vi "nanocal -- nuclear schottky fit V8.vi"() -> ()   [LabVIEW 2021] (continued)
  out "string OUT":string="  \"IDS0158_210310_RAW_cal__ref_\" ->   <|    \"ζ\" -> 0.342934102355   ,  \"τ1\" -> 0.037912336866   ,  \"τS\" -> 0.322770587290   ,  \"τN\" -> 0.224517468406   ,  \"τC\" -> 0.000970428995   ,  \"κ0\" -> 0.000000000517   ,  \"mm1\" -> 0.000247395955   ,  \"mm2\" -> 0.021898106728   ,  \"mm3\" -> 0.751709056984   ,  \"T\" -> 0.120000000000   ,  \"B\" -> 12.000000000000   ,  \"θ\" -> 0.000000000000   ,  \"Reoff\" -> 0.000000000000   ,  \"Imoff\" -> 0.000000000000   ,  \"στ1\" -> 0.000893425914   ,  \"στS\" -> 0.002489408176   ,  \"στN\" -> 0.002611842121   ,  \"τ11 \" -> 0.000000000000   ,  \"τ12\" -> 0.000000000000   ,  \"τ22\" -> 0.000000000000   ,  \"τN1\" -> 0.000000000000   ,  \"τN2\" -> 0.000000000000   ,  \"σηlogτ1 \" -> 0.114569772809   ,  \"σηlogτS\" -> 0.007573309274   ,  \"σηlogτN\" -> 0.068166495911   ,  \"σlogτ1\" -> 0.023565572257   ,  \"σlogτS\" -> 0.007712623993   ,  \"σlogτN\" -> 0.011633135451   ,  \"σητ1\" -> 0.004343607821   ,  \"σητS \" -> 0.002444441482   ,  \"σητN\" -> 0.015304569092    |>   , \r\"IDS0158_210310_RAW_cal__sam_\" ->   <|    \"ζ\" -> 0.286336668596   ,  \"τ1\" -> 0.037477267671   ,  \"τS\" -> 0.354459287884   ,  \"τN\" -> 0.444916383639   ,  \"τC\" -> 0.001225600579   ,  \"κ0\" -> 0.000000000596   ,  \"mm1\" -> 0.000272242393   ,  \"mm2\" -> 0.016302418461   ,  \"mm3\" -> 1.050394445660   ,  \"T\" -> 0.120000000000   ,  \"B\" -> 12.000000000000   ,  \"θ\" -> 0.000000000000   ,  \"Reoff\" -> 0.000000000000   ,  \"Imoff\" -> 0.000000000000   ,  \"στ1\" -> 0.000000000000   ,  \"στS\" -> 0.000000000000   ,  \"στN\" -> 0.000000000000   ,  \"τ11 \" -> 0.000000000000   ,  \"τ12\" -> 0.000000000000   ,  \"τ22\" -> 0.000000000000   ,  \"τN1\" -> 0.000000000000   ,  \"τN2\" -> 0.000000000000   ,  \"σηlogτ1 \" -> 0.000000000000   ,  \"σηlogτS\" -> 0.000000000000   ,  \"σηlogτN\" -> 0.000000000000   ,  \"σlogτ1\" -> 0.000000000000   ,  \"σlogτS\" -> 0.000000000000   ,  \"σlogτN\" -> 0.000000000000   ,  \"σητ1\" -> 0.000000000000   ,  \"σητS \" -> 0.000000000000   ,  \"σητN\" -> 0.000000000000    |>   , \r\"IDS0159_210310_RAW_cal__ref_\" ->   <|    \"ζ\" -> 0.271761862806   ,  \"τ1\" -> 0.039955104592   ,  \"τS\" -> 0.227503722031   ,  \"τN\" -> 0.142080712192   ,  \"τC\" -> 0.000995450305   ,  \"κ0\" -> 0.000000000652   ,  \"mm1\" -> 0.000212140795   ,  \"mm2\" -> 0.023804196565   ,  \"mm3\" -> 0.486957606069   ,  \"T\" -> 0.150000000000   ,  \"B\" -> 12.000000000000   ,  \"θ\" -> 0.000000000000   ,  \"Reoff\" -> 0.000000000000   ,  \"Imoff\" -> 0.000000000000   ,  \"στ1\" -> 0.000698593116   ,  \"στS\" -> 0.001142949493   ,  \"στN\" -> 0.001230291496   ,  \"τ11 \" -> 0.000000000000   ,  \"τ12\" -> 0.000000000000   ,  \"τ22\" -> 0.000000000000   ,  \"τN1\" -> 0.000000000000   ,  \"τN2\" -> 0.000000000000   ,  \"σηlogτ1 \" -> 0.100498796621   ,  \"σηlogτS\" -> 0.005660617730   ,  \"σηlogτN\" -> 0.063140982058   ,  \"σlogτ1\" -> 0.017484452181   ,  \"σlogτS\" -> 0.005023871622   ,  \"σlogτN\" -> 0.008659102821   ,  \"σητ1\" -> 0.004015439930   ,  \"σητS \" -> 0.001287811603   ,  \"σητN\" -> 0.008971115699    |>   , \r\"IDS0159_210310_RAW_cal__sam_\" ->   <|    \"ζ\" -> 0.219100303741   ,  \"τ1\" -> 0.028643012604   ,  \"τS\" -> 0.279362928811   ,  \"τN\" -> 0.246156444058   ,  \"τC\" -> 0.001272401549   ,  \"κ0\" -> 0.000000000760   ,  \"mm1\" -> 0.000227975653   ,  \"mm2\" -> 0.014929571562   ,  \"mm3\" -> 0.655418694024   ,  \"T\" -> 0.150000000000   ,  \"B\" -> 12.000000000000   ,  \"θ\" -> 0.000000000000   ,  \"Reoff\" -> 0.000000000000   ,  \"Imoff\" -> 0.000000000000   ,  \"στ1\" -> 0.000000000000   ,  \"στS\" -> 0.000000000000   ,  \"στN\" -> 0.000000000000   ,  \"τ11 \" -> 0.000000000000   ,  \"τ12\" -> 0.000000000000   ,  \"τ22\" -> 0.000000000000   ,  \"τN1\" -> 0.000000000000   ,  \"τN2\" -> 0.000000000000   ,  \"σηlogτ1 \" -> 0.000000000000   ,  \"σηlogτS\" -> 0.000000000000   ,  \"σηlogτN\" -> 0.000000000000   ,  \"σlogτ1\" -> 0.000000000000   ,  \"σlogτS\" -> 0.000000000000   ,  \"σlogτN\" -> 0.000000000000   ,  \"σητ1\" -> 0.000000000000   ,  \"σητS \" -> 0.000000000000   ,  \"σητN\" -> 0.000000000000    |>   , \r\"IDS0160_210310_RAW_cal__ref_\" ->   <|    \"ζ\" -> 0.199613086212   ,  \"τ1\" -> 0.022193731398   ,  \"τS\" -> 0.116862561742   ,  \"τN\" -> 0.097247059130   ,  \"τC\" -> 0.001045881960   ,  \"κ0\" -> 0.000000000931   ,  \"mm1\" -> 0.000172948552   ,  \"mm2\" -> 0.011671612475   ,  \"mm3\" -> 0.268243755414   ,  \"T\" -> 0.180000000000   ,  \"B\" -> 12.000000000000   ,  \"θ\" -> 0.000000000000   ,  \"Reoff\" -> 0.000000000000   ,  \"Imoff\" -> 0.000000000000   ,  \"στ1\" -> 0.000089856815   ,  \"στS\" -> 0.000165029214   ,  \"στN\" -> 0.000188286128   ,  \"τ11 \" -> 0.000000000000   ,  \"τ12\" -> 0.000000000000   ,  \"τ22\" -> 0.000000000000   ,  \"τN1\" -> 0.000000000000   ,  \"τN2\" -> 0.000000000000   ,  \"σηlogτ1 \" -> 0.093550953866   ,  \"σηlogτS\" -> 0.006075230131   ,  \"σηlogτN\" -> 0.064015363974   ,  \"σlogτ1\" -> 0.004048747519   ,  \"σlogτS\" -> 0.001412164955   ,  \"σlogτN\" -> 0.001936162698   ,  \"σητ1\" -> 0.002076244742   ,  \"σητS \" -> 0.000709966956   ,  \"σητN\" -> 0.006225305886    |>   , \r\"IDS0160_210310_RAW_cal__sam_\" ->   <|    \"ζ\" -> 0.170488637524   ,  \"τ1\" -> 0.029234231120   ,  \"τS\" -> 0.149095458227   ,  \"τN\" -> 0.151792620275   ,  \"τC\" -> 0.001113424175   ,  \"κ0\" -> 0.000000001042   ,  \"mm1\" -> 0.000161291869   ,  \"mm2\" -> 0.013922632736   ,  \"mm3\" -> 0.368449807743   ,  \"T\" -> 0.180000000000   ,  \"B\" -> 12.000000000000   ,  \"θ\" -> 0.000000000000   ,  \"Reoff\" -> 0.000000000000   ,  \"Imoff\" -> 0.000000000000   ,  \"στ1\" -> 0.000000000000   ,  \"στS\" -> 0.000000000000   ,  \"στN\" -> 0.000000000000   ,  \"τ11 \" -> 0.000000000000   ,  \"τ12\" -> 0.000000000000   ,  \"τ22\" -> 0.000000000000   ,  \"τN1\" -> 0.000000000000   ,  \"τN2\" -> 0.000000000000   ,  \"σηlogτ1 \" -> 0.000000000000   ,  \"σηlogτS\" -> 0.000000000000   ,  \"σηlogτN\" -> 0.000000000000   ,  \"σlogτ1\" -> 0.000000000000   ,  \"σlogτS\" -> 0.000000000000   ,  \"σlogτN\" -> 0.000000000000   ,  \"σητ1\" -> 0.000000000000   ,  \"σητS \" -> 0.000000000000   ,  \"σητN\" -> 0.000000000000    |>   , \r\"IDS0161_210310_RAW_cal__ref_\" ->   <|    \"ζ\" -> 0.155485326727   ,  \"τ1\" -> 0.024589160211   ,  \"τS\" -> 0.103187251839   ,  \"τN\" -> 0.059327264902   ,  \"τC\" -> 0.001362397594   ,  \"κ0\" -> 0.000000001075   ,  \"mm1\" -> 0.000181522487   ,  \"mm2\" -> 0.014905594718   ,  \"mm3\" -> 0.198647580074   ,  \"T\" -> 0.200000000000   ,  \"B\" -> 12.000000000000   ,  \"θ\" -> 0.000000000000   ,  \"Reoff\" -> 0.000000000000   ,  \"Imoff\" -> 0.000000000000   ,  \"στ1\" -> 0.000106824093   ,  \"στS\" -> 0.000114207069   ,  \"στN\" -> 0.000127738509   ,  \"τ11 \" -> 0.000000000000   ,  \"τ12\" -> 0.000000000000   ,  \"τ22\" -> 0.000000000000   ,  \"τN1\" -> 0.000000000000   ,  \"τN2\" -> 0.000000000000   ,  \"σηlogτ1 \" -> 0.086294510505   ,  \"σηlogτS\" -> 0.004144737065   ,  \"σηlogτN\" -> 0.058529518145   ,  \"σlogτ1\" -> 0.004344357106   ,  \"σlogτS\" -> 0.001106794371   ,  \"σlogτN\" -> 0.002153116435   ,  \"σητ1\" -> 0.002121909544   ,  \"σητS \" -> 0.000427684027   ,  \"σητN\" -> 0.003472396228    |>   , \r\"IDS0161_210310_RAW_cal__sam_\" ->   <|    \"ζ\" -> 0.130531197151   ,  \"τ1\" -> 0.025704482770   ,  \"τS\" -> 0.129606657196   ,  \"τN\" -> 0.091602369165   ,  \"τC\" -> 0.001441379995   ,  \"κ0\" -> 0.000000001211   ,  \"mm1\" -> 0.000164978070   ,  \"mm2\" -> 0.014468182937   ,  \"mm3\" -> 0.262596407151   ,  \"T\" -> 0.200000000000   ,  \"B\" -> 12.000000000000   ,  \"θ\" -> 0.000000000000   ,  \"Reoff\" -> 0.000000000000   ,  \"Imoff\" -> 0.000000000000   ,  \"στ1\" -> 0.000000000000   ,  \"στS\" -> 0.000000000000   ,  \"στN\" -> 0.000000000000   ,  \"τ11 \" -> 0.000000000000   ,  \"τ12\" -> 0.000000000000   ,  \"τ22\" -> 0.000000000000   ,  \"τN1\" -> 0.000000000000   ,  \"τN2\" -> 0.000000000000   ,  \"σηlogτ1 \" -> 0.000000000000   ,  \"σηlogτS\" -> 0.000000000000   ,  \"σηlogτN\" -> 0.000000000000   ,  \"σlogτ1\" -> 0.000000000000   ,  \"σlogτS\" -> 0.000000000000   ,  \"σlogτN\" -> 0.000000000000   ,  \"σητ1\" -> 0.000000000000   ,  \"σητS \" -> 0.000000000000   ,  \"σητN\" -> 0.000000000000    |>   , \r\"IDS0162_210310_RAW_cal__ref_\" ->   <|    \"ζ\" -> 0.085932974943   ,  \"τ1\" -> 0.018822470857   ,  \"τS\" -> 0.068810147904   ,  \"τN\" -> 0.024216831887   ,  \"τC\" -> 0.001953952621   ,  \"κ0\" -> 0.000000001388   ,  \"mm1\" -> 0.000150968751   ,  \"mm2\" -> 0.013294741414   ,  \"mm3\" -> 0.108351778227   ,  \"T\" -> 0.250000000000   ,  \"B\" -> 12.000000000000   ,  \"θ\" -> 0.000000000000   ,  \"Reoff\" -> 0.000000000000   ,  \"Imoff\" -> 0.000000000000   ,  \"στ1\" -> 0.000058321163   ,  \"στS\" -> 0.000035049706   ,  \"στN\" -> 0.000037861271   ,  \"τ11 \" -> 0.000000000000   ,  \"τ12\" -> 0.000000000000   ,  \"τ22\" -> 0.000000000000   ,  \"τN1\" -> 0.000000000000   ,  \"τN2\" -> 0.000000000000   ,  \"σηlogτ1 \" -> 0.080513059924   ,  \"σηlogτS\" -> 0.002518022810   ,  \"σηlogτN\" -> 0.054257654253   ,  \"σlogτ1\" -> 0.003098486056   ,  \"σlogτS\" -> 0.000509368271   ,  \"σlogτN\" -> 0.001563427918   ,  \"σητ1\" -> 0.001515454724   ,  \"σητS \" -> 0.000173265522   ,  \"σητN\" -> 0.001313948492    |>   , \r\"IDS0162_210310_RAW_cal__sam_\" ->   <|    \"ζ\" -> 0.078258046754   ,  \"τ1\" -> 0.028009840731   ,  \"τS\" -> 0.092122038762   ,  \"τN\" -> 0.030129595899   ,  \"τC\" -> 0.001641062244   ,  \"κ0\" -> 0.000000001543   ,  \"mm1\" -> 0.000117303440   ,  \"mm2\" -> 0.019983073008   ,  \"mm3\" -> 0.141369335330   ,  \"T\" -> 0.250000000000   ,  \"B\" -> 12.000000000000   ,  \"θ\" -> 0.000000000000   ,  \"Reoff\" -> 0.000000000000   ,  \"Imoff\" -> 0.000000000000   ,  \"στ1\" -> 0.000000000000   ,  \"στS\" -> 0.000000000000   ,  \"στN\" -> 0.000000000000   ,  \"τ11 \" -> 0.000000000000   ,  \"τ12\" -> 0.000000000000   ,  \"τ22\" -> 0.000000000000   ,  \"τN1\" -> 0.000000000000   ,  \"τN2\" -> 0.000000000000   ,  \"σηlogτ1 \" -> 0.000000000000   ,  \"σηlogτS\" -> 0.000000000000   ,  \"σηlogτN\" -> 0.000000000000   ,  \"σlogτ1\" -> 0.000000000000   ,  \"σlogτS\" -> 0.000000000000   ,  \"σlogτN\" -> 0.000000000000   ,  \"σητ1\" -> 0.000000000000   ,  \"σητS \" -> 0.000000000000   ,  \"σητN\" -> 0.000000000000    |>   , \r\"IDS0163_210310_RAW_cal__ref_\" ->   <|    \"ζ\" -> 0.058825748663   ,  \"τ1\" -> 0.015012107932   ,  \"τS\" -> 0.052128918860   ,  \"τN\" -> 0.012953217864   ,  \"τC\" -> 0.002393557537   ,  \"κ0\" -> 0.000000001766   ,  \"mm1\" -> 0.000127725677   ,  \"mm2\" -> 0.011559700576   ,  \"mm3\" -> 0.074628881357   ,  \"T\" -> 0.300000000000   ,  \"B\" -> 12.000000000000   ,  \"θ\" -> 0.000000000000   ,  \"Reoff\" -> 0.000000000000   ,  \"Imoff\" -> 0.000000000000   ,  \"στ1\" -> 0.000023064935   ,  \"στS\" -> 0.000009573131   ,  \"στN\" -> 0.000010092664   ,  \"τ11 \" -> 0.000000000000   ,  \"τ12\" -> 0.000000000000   ,  \"τ22\" -> 0.000000000000   ,  \"τN1\" -> 0.000000000000   ,  \"τN2\" -> 0.000000000000   ,  \"σηlogτ1 \" -> 0.078709092172   ,  \"σηlogτS\" -> 0.001802886041   ,  \"σηlogτN\" -> 0.052574057148   ,  \"σlogτ1\" -> 0.001536422126   ,  \"σlogτS\" -> 0.000183643382   ,  \"σlogτN\" -> 0.000779162669   ,  \"σητ1\" -> 0.001181589387   ,  \"σητS \" -> 0.000093982500   ,  \"σητN\" -> 0.000681003216    |>   , \r\"IDS0163_210310_RAW_cal__sam_\" ->   <|    \"ζ\" -> 0.054088186012   ,  \"τ1\" -> 0.023838802615   ,  \"τS\" -> 0.069079396629   ,  \"τN\" -> 0.016435267456   ,  \"τC\" -> 0.002025071743   ,  \"κ0\" -> 0.000000001955   ,  \"mm1\" -> 0.000101234646   ,  \"mm2\" -> 0.018244822177   ,  \"mm3\" -> 0.097657814678   ,  \"T\" -> 0.300000000000   ,  \"B\" -> 12.000000000000   ,  \"θ\" -> 0.000000000000   ,  \"Reoff\" -> 0.000000000000   ,  \"Imoff\" -> 0.000000000000   ,  \"στ1\" -> 0.000000000000   ,  \"στS\" -> 0.000000000000   ,  \"στN\" -> 0.000000000000   ,  \"τ11 \" -> 0.000000000000   ,  \"τ12\" -> 0.000000000000   ,  \"τ22\" -> 0.000000000000   ,  \"τN1\" -> 0.000000000000   ,  \"τN2\" -> 0.000000000000   ,  \"σηlogτ1 \" -> 0.000000000000   ,  \"σηlogτS\" -> 0.000000000000   ,  \"σηlogτN\" -> 0.000000000000   ,  \"σlogτ1\" -> 0.000000000000   ,  \"σlogτS\" -> 0.000000000000   ,  \"σlogτN\" -> 0.000000000000   ,  \"σητ1\" -> 0.000000000000   ,  \"σητS \" -> 0.000000000000   ,  \"σητN\" -> 0.000000000000    |>   , \r\"IDS0164_210310_RAW_cal__ref_\" ->   <|    \"ζ\" -> 0.042805749253   ,  \"τ1\" -> 0.013206199214   ,  \"τS\" -> 0.042245691100   ,  \"τN\" -> 0.007144228501   ,  \"τC\" -> 0.002899499229   ,  \"κ0\" -> 0.000000002181   ,  \"mm1\" -> 0.000111927858   ,  \"mm2\" -> 0.010938028304   ,  \"mm3\" -> 0.056559834396   ,  \"T\" -> 0.360000000000   ,  \"B\" -> 12.000000000000   ,  \"θ\" -> 0.000000000000   ,  \"Reoff\" -> 0.000000000000   ,  \"Imoff\" -> 0.000000000000   ,  \"στ1\" -> 0.000012292384   ,  \"στS\" -> 0.000003241338   ,  \"στN\" -> 0.000003368378   ,  \"τ11 \" -> 0.000000000000   ,  \"τ12\" -> 0.000000000000   ,  \"τ22\" -> 0.000000000000   ,  \"τN1\" -> 0.000000000000   ,  \"τN2\" -> 0.000000000000   ,  \"σηlogτ1 \" -> 0.075974060792   ,  \"σηlogτS\" -> 0.001194926073   ,  \"σηlogτN\" -> 0.051138297484   ,  \"σlogτ1\" -> 0.000930804037   ,  \"σlogτS\" -> 0.000076725884   ,  \"σlogτN\" -> 0.000471482447   ,  \"σητ1\" -> 0.001003328582   ,  \"σητS \" -> 0.000050480478   ,  \"σητN\" -> 0.000365343682    |>   , \r\"IDS0164_210310_RAW_cal__sam_\" ->   <|    \"ζ\" -> 0.039314966212   ,  \"τ1\" -> 0.020712803909   ,  \"τS\" -> 0.055413767550   ,  \"τN\" -> 0.008474403424   ,  \"τC\" -> 0.002674063387   ,  \"κ0\" -> 0.000000002415   ,  \"mm1\" -> 0.000096818147   ,  \"mm2\" -> 0.017190811405   ,  \"mm3\" -> 0.072499170001   ,  \"T\" -> 0.360000000000   ,  \"B\" -> 12.000000000000   ,  \"θ\" -> 0.000000000000   ,  \"Reoff\" -> 0.000000000000   ,  \"Imoff\" -> 0.000000000000   ,  \"στ1\" -> 0.000000000000   ,  \"στS\" -> 0.000000000000   ,  \"στN\" -> 0.000000000000   ,  \"τ11 \" -> 0.000000000000   ,  \"τ12\" -> 0.000000000000   ,  \"τ22\" -> 0.000000000000   ,  \"τN1\" -> 0.000000000000   ,  \"τN2\" -> 0.000000000000   ,  \"σηlogτ1 \" -> 0.000000000000   ,  \"σηlogτS\" -> 0.000000000000   ,  \"σηlogτN\" -> 0.000000000000   ,  \"σlogτ1\" -> 0.000000000000   ,  \"σlogτS\" -> 0.000000000000   ,  \"σlogτN\" -> 0.000000000000   ,  \"σητ1\" -> 0.000000000000   ,  \"σητS \" -> 0.000000000000   ,  \"σητN\" -> 0.000000000000    |>   , \r\"IDS0165_210310_RAW_cal__ref_\" ->   <|    \"ζ\" -> 0.032274621211   ,  \"τ1\" -> 0.011425652621   ,  \"τS\" -> 0.034817148793   ,  \"τN\" -> 0.004293407669   ,  \"τC\" -> 0.003209213512   ,  \"κ0\" -> 0.000000002697   ,  \"mm1\" -> 0.000092323212   ,  \"mm2\" -> 0.009918344751   ,  \"mm3\" -> 0.044997033026   ,  \"T\" -> 0.430000000000   ,  \"B\" -> 12.000000000000   ,  \"θ\" -> 0.000000000000   ,  \"Reoff\" -> 0.000000000000   ,  \"Imoff\" -> 0.000000000000   ,  \"στ1\" -> 0.000021533973   ,  \"στS\" -> 0.000003977444   ,  \"στN\" -> 0.000004093454   ,  \"τ11 \" -> 0.000000000000   ,  \"τ12\" -> 0.000000000000   ,  \"τ22\" -> 0.000000000000   ,  \"τN1\" -> 0.000000000000   ,  \"τN2\" -> 0.000000000000   ,  \"σηlogτ1 \" -> 0.074657261466   ,  \"σηlogτS\" -> 0.000861446772   ,  \"σηlogτN\" -> 0.050403269276   ,  \"σlogτ1\" -> 0.001884703953   ,  \"σlogτS\" -> 0.000114238081   ,  \"σlogτN\" -> 0.000953427722   ,  \"σητ1\" -> 0.000853007935   ,  \"σητS \" -> 0.000029993120   ,  \"σητN\" -> 0.000216401783    |>   , \r\"IDS0165_210310_RAW_cal__sam_\" ->   <|    \"ζ\" -> 0.031945976845   ,  \"τ1\" -> 0.019000922826   ,  \"τS\" -> 0.045624146388   ,  \"τN\" -> 0.005314716063   ,  \"τC\" -> 0.002488383471   ,  \"κ0\" -> 0.000000002954   ,  \"mm1\" -> 0.000073272643   ,  \"mm2\" -> 0.016306894362   ,  \"mm3\" -> 0.057675293464   ,  \"T\" -> 0.430000000000   ,  \"B\" -> 12.000000000000   ,  \"θ\" -> 0.000000000000   ,  \"Reoff\" -> 0.000000000000   ,  \"Imoff\" -> 0.000000000000   ,  \"στ1\" -> 0.000000000000   ,  \"στS\" -> 0.000000000000   ,  \"στN\" -> 0.000000000000   ,  \"τ11 \" -> 0.000000000000   ,  \"τ12\" -> 0.000000000000   ,  \"τ22\" -> 0.000000000000   ,  \"τN1\" -> 0.000000000000   ,  \"τN2\" -> 0.000000000000   ,  \"σηlogτ1 \" -> 0.000000000000   ,  \"σηlogτS\" -> 0.000000000000   ,  \"σηlogτN\" -> 0.000000000000   ,  \"σlogτ1\" -> 0.000000000000   ,  \"σlogτS\" -> 0.000000000000   ,  \"σlogτN\" -> 0.000000000000   ,  \"σητ1\" -> 0.000000000000   ,  \"σητS \" -> 0.000000000000   ,  \"σητN\" -> 0.000000000000    |>   , \r\"IDS0166_210310_RAW_cal__ref_\" ->   <|    \"ζ\" -> 0.024856483242   ,  \"τ1\" -> 0.010695421072   ,  \"τS\" -> 0.028584689386   ,  \"τN\" -> 0.002299338912   ,  \"τC\" -> 0.003707358018   ,  \"κ0\" -> 0.000000003388   ,  \"mm1\" -> 0.000080004626   ,  \"mm2\" -> 0.009710607688   ,  \"mm3\" -> 0.036263863406   ,  \"T\" -> 0.520000000000   ,  \"B\" -> 12.000000000000   ,  \"θ\" -> 0.000000000000   ,  \"Reoff\" -> 0.000000000000   ,  \"Imoff\" -> 0.000000000000   ,  \"στ1\" -> 0.000044725972   ,  \"στS\" -> 0.000004660348   ,  \"στN\" -> 0.000004819065   ,  \"τ11 \" -> 0.000000000000   ,  \"τ12\" -> 0.000000000000   ,  \"τ22\" -> 0.000000000000   ,  \"τN1\" -> 0.000000000000   ,  \"τN2\" -> 0.000000000000   ,  \"σηlogτ1 \" -> 0.070445110801   ,  \"σηlogτS\" -> 0.000510235434   ,  \"σηlogτN\" -> 0.049344443023   ,  \"σlogτ1\" -> 0.004181786915   ,  \"σlogτS\" -> 0.000163036495   ,  \"σlogτN\" -> 0.002095848078   ,  \"σητ1\" -> 0.000753440123   ,  \"σητS \" -> 0.000014584921   ,  \"σητN\" -> 0.000113459598    |>   , \r\"IDS0166_210310_RAW_cal__sam_\" ->   <|    \"ζ\" -> 0.023031239946   ,  \"τ1\" -> 0.018268814012   ,  \"τS\" -> 0.037269400776   ,  \"τN\" -> 0.002696792890   ,  \"τC\" -> 0.003257395394   ,  \"κ0\" -> 0.000000003720   ,  \"mm1\" -> 0.000067670174   ,  \"mm2\" -> 0.016445281937   ,  \"mm3\" -> 0.045899921957   ,  \"T\" -> 0.520000000000   ,  \"B\" -> 12.000000000000   ,  \"θ\" -> 0.000000000000   ,  \"Reoff\" -> 0.000000000000   ,  \"Imoff\" -> 0.000000000000   ,  \"στ1\" -> 0.000000000000   ,  \"στS\" -> 0.000000000000   ,  \"στN\" -> 0.000000000000   ,  \"τ11 \" -> 0.000000000000   ,  \"τ12\" -> 0.000000000000   ,  \"τ22\" -> 0.000000000000   ,  \"τN1\" -> 0.000000000000   ,  \"τN2\" -> 0.000000000000   ,  \"σηlogτ1 \" -> 0.000000000000   ,  \"σηlogτS\" -> 0.000000000000   ,  \"σηlogτN\" -> 0.000000000000   ,  \"σlogτ1\" -> 0.000000000000   ,  \"σlogτS\" -> 0.000000000000   ,  \"σlogτN\" -> 0.000000000000   ,  \"σητ1\" -> 0.000000000000   ,  \"σητS \" -> 0.000000000000   ,  \"σητN\" -> 0.000000000000    |>   , \r\"IDS0167_210310_RAW_cal__ref_\" ->   <|    \"ζ\" -> 0.023755086775   ,  \"τ1\" -> 0.012442537684   ,  \"τS\" -> 0.025226466021   ,  \"τN\" -> 0.001327754553   ,  \"τC\" -> 0.003535029288   ,  \"κ0\" -> 0.000000003992   ,  \"mm1\" -> 0.000072325961   ,  \"mm2\" -> 0.011557286901   ,  \"mm3\" -> 0.031532972498   ,  \"T\" -> 0.620000000000   ,  \"B\" -> 12.000000000000   ,  \"θ\" -> 0.000000000000   ,  \"Reoff\" -> 0.000000000000   ,  \"Imoff\" -> 0.000000000000   ,  \"στ1\" -> 0.000121120374   ,  \"στS\" -> 0.000005759367   ,  \"στN\" -> 0.000006380048   ,  \"τ11 \" -> 0.000000000000   ,  \"τ12\" -> 0.000000000000   ,  \"τ22\" -> 0.000000000000   ,  \"τN1\" -> 0.000000000000   ,  \"τN2\" -> 0.000000000000   ,  \"σηlogτ1 \" -> 0.060087437694   ,  \"σηlogτS\" -> 0.000239286620   ,  \"σηlogτN\" -> 0.047627856995   ,  \"σlogτ1\" -> 0.009734378741   ,  \"σlogτS\" -> 0.000228306534   ,  \"σlogτN\" -> 0.004805140830   ,  \"σητ1\" -> 0.000747640208   ,  \"σητS \" -> 0.000006036356   ,  \"σητN\" -> 0.000063238104    |>   , \r\"IDS0167_210310_RAW_cal__sam_\" ->   <|    \"ζ\" -> 0.019920170845   ,  \"τ1\" -> 0.016368892412   ,  \"τS\" -> 0.030579536580   ,  \"τN\" -> 0.001736017565   ,  \"τC\" -> 0.004971418152   ,  \"κ0\" -> 0.000000004410   ,  \"mm1\" -> 0.000083939556   ,  \"mm2\" -> 0.015095997595   ,  \"mm3\" -> 0.039119658918   ,  \"T\" -> 0.620000000000   ,  \"B\" -> 12.000000000000   ,  \"θ\" -> 0.000000000000   ,  \"Reoff\" -> 0.000000000000   ,  \"Imoff\" -> 0.000000000000   ,  \"στ1\" -> 0.000000000000   ,  \"στS\" -> 0.000000000000   ,  \"στN\" -> 0.000000000000   ,  \"τ11 \" -> 0.000000000000   ,  \"τ12\" -> 0.000000000000   ,  \"τ22\" -> 0.000000000000   ,  \"τN1\" -> 0.000000000000   ,  \"τN2\" -> 0.000000000000   ,  \"σηlogτ1 \" -> 0.000000000000   ,  \"σηlogτS\" -> 0.000000000000   ,  \"σηlogτN\" -> 0.000000000000   ,  \"σlogτ1\" -> 0.000000000000   ,  \"σlogτS\" -> 0.000000000000   ,  \"σlogτN\" -> 0.000000000000   ,  \"σητ1\" -> 0.000000000000   ,  \"σητS \" -> 0.000000000000   ,  \"σητN\" -> 0.000000000000    |>   , \r\"IDS0168_210310_RAW_cal__ref_\" ->   <|    \"ζ\" -> 0.018175201883   ,  \"τ1\" -> 0.013383195137   ,  \"τS\" -> 0.017675939869   ,  \"τN\" -> 0.000584160710   ,  \"τC\" -> 0.005568397021   ,  \"κ0\" -> 0.000000005579   ,  \"mm1\" -> 0.000076155273   ,  \"mm2\" -> 0.012686054664   ,  \"mm3\" -> 0.024781363815   ,  \"T\" -> 0.810000000000   ,  \"B\" -> 12.000000000000   ,  \"θ\" -> 0.000000000000   ,  \"Reoff\" -> 0.000000000000   ,  \"Imoff\" -> 0.000000000000   ,  \"στ1\" -> 0.000105801087   ,  \"στS\" -> 0.000001832616   ,  \"στN\" -> 0.000002314917   ,  \"τ11 \" -> 0.000000000000   ,  \"τ12\" -> 0.000000000000   ,  \"τ22\" -> 0.000000000000   ,  \"τN1\" -> 0.000000000000   ,  \"τN2\" -> 0.000000000000   ,  \"σηlogτ1 \" -> 0.050518101739   ,  \"σηlogτS\" -> 0.000100664856   ,  \"σηlogτN\" -> 0.045919539288   ,  \"σlogτ1\" -> 0.007905517739   ,  \"σlogτS\" -> 0.000103678550   ,  \"σlogτN\" -> 0.003962808035   ,  \"σητ1\" -> 0.000676093614   ,  \"σητS \" -> 0.000001779346   ,  \"σητN\" -> 0.000026824391    |>   , \r\"IDS0168_210310_RAW_cal__sam_\" ->   <|    \"ζ\" -> 0.017558473054   ,  \"τ1\" -> 0.014545104284   ,  \"τS\" -> 0.022979681288   ,  \"τN\" -> 0.000840829385   ,  \"τC\" -> 0.005228030240   ,  \"κ0\" -> 0.000000006068   ,  \"mm1\" -> 0.000073916527   ,  \"mm2\" -> 0.013750428362   ,  \"mm3\" -> 0.030187552103   ,  \"T\" -> 0.810000000000   ,  \"B\" -> 12.000000000000   ,  \"θ\" -> 0.000000000000   ,  \"Reoff\" -> 0.000000000000   ,  \"Imoff\" -> 0.000000000000   ,  \"στ1\" -> 0.000000000000   ,  \"στS\" -> 0.000000000000   ,  \"στN\" -> 0.000000000000   ,  \"τ11 \" -> 0.000000000000   ,  \"τ12\" -> 0.000000000000   ,  \"τ22\" -> 0.000000000000   ,  \"τN1\" -> 0.000000000000   ,  \"τN2\" -> 0.000000000000   ,  \"σηlogτ1 \" -> 0.000000000000   ,  \"σηlogτS\" -> 0.000000000000   ,  \"σηlogτN\" -> 0.000000000000   ,  \"σlogτ1\" -> 0.000000000000   ,  \"σlogτS\" -> 0.000000000000   ,  \"σlogτN\" -> 0.000000000000   ,  \"σητ1\" -> 0.000000000000   ,  \"σητS \" -> 0.000000000000   ,  \"σητN\" -> 0.000000000000    |>   , \r\"IDS0169_210310_RAW_cal__ref_\" ->   <|    \"ζ\" -> 0.019957179421   ,  \"τ1\" -> 0.013979356395   ,  \"τS\" -> 0.014979933171   ,  \"τN\" -> 0.000246381668   ,  \"τC\" -> 0.003917957379   ,  \"κ0\" -> 0.000000007787   ,  \"mm1\" -> 0.000061209589   ,  \"mm2\" -> 0.013393834195   ,  \"mm3\" -> 0.019972459127   ,  \"T\" -> 1.120000000000   ,  \"B\" -> 12.000000000000   ,  \"θ\" -> 0.000000000000   ,  \"Reoff\" -> -604081.632653061067   ,  \"Imoff\" -> 0.000000000000   ,  \"στ1\" -> 0.016865078301   ,  \"στS\" -> 0.000159497722   ,  \"στN\" -> 0.007867947468   ,  \"τ11 \" -> 0.000000000000   ,  \"τ12\" -> 0.000000000000   ,  \"τ22\" -> 0.000000000000   ,  \"τN1\" -> 0.000000000000   ,  \"τN2\" -> 0.000000000000   ,  \"σηlogτ1 \" -> 0.000000000000   ,  \"σηlogτS\" -> 0.000000000000   ,  \"σηlogτN\" -> 0.000000000000   ,  \"σlogτ1\" -> 0.000000000000   ,  \"σlogτS\" -> 0.000000000000   ,  \"σlogτN\" -> 0.000000000000   ,  \"σητ1\" -> 0.000000000000   ,  \"σητS \" -> 0.000000000000   ,  \"σητN\" -> 0.000000000000    |>   , \r\"IDS0169_210310_RAW_cal__sam_\" ->   <|    \"ζ\" -> 0.011916480594   ,  \"τ1\" -> 0.012551282481   ,  \"τS\" -> 0.018233218660   ,  \"τN\" -> 0.000345702746   ,  \"τC\" -> 0.004699451527   ,  \"κ0\" -> 0.000000008451   ,  \"mm1\" -> 0.000044190864   ,  \"mm2\" -> 0.012162820727   ,  \"mm3\" -> 0.023844039179   ,  \"T\" -> 1.120000000000   ,  \"B\" -> 12.000000000000   ,  \"θ\" -> 0.000000000000   ,  \"Reoff\" -> 0.000000000000   ,  \"Imoff\" -> 0.000000000000   ,  \"στ1\" -> 0.000000000000   ,  \"στS\" -> 0.000000000000   ,  \"στN\" -> 0.000000000000   ,  \"τ11 \" -> 0.000000000000   ,  \"τ12\" -> 0.000000000000   ,  \"τ22\" -> 0.000000000000   ,  \"τN1\" -> 0.000000000000   ,  \"τN2\" -> 0.000000000000   ,  \"σηlogτ1 \" -> 0.000000000000   ,  \"σηlogτS\" -> 0.000000000000   ,  \"σηlogτN\" -> 0.000000000000   ,  \"σlogτ1\" -> 0.000000000000   ,  \"σlogτS\" -> 0.000000000000   ,  \"σlogτN\" -> 0.000000000000   ,  \"σητ1\" -> 0.000000000000   ,  \"σητS \" -> 0.000000000000   ,  \"σητN\" -> 0.000000000000    |>   , \r\"IDS0170_210310_RAW_cal__ref_\" ->   <|    \"ζ\" -> 0.020917521423   ,  \"τ1\" -> 0.014571936752   ,  \"τS\" -> 0.010774968577   ,  \"τN\" -> 0.000062073801   ,  \"τC\" -> 0.003888097391   ,  \"κ0\" -> 0.000000012613   ,  \"mm1\" -> 0.000059093319   ,  \"mm2\" -> 0.013758745196   ,  \"mm3\" -> 0.015705922073   ,  \"T\" -> 1.800000000000   ,  \"B\" -> 12.000000000000   ,  \"θ\" -> 0.000000000000   ,  \"Reoff\" -> -530612.244897959054   ,  \"Imoff\" -> 0.000000000000   ,  \"στ1\" -> 0.055735786157   ,  \"στS\" -> 0.000157216248   ,  \"στN\" -> 0.024225134913   ,  \"τ11 \" -> 0.000000000000   ,  \"τ12\" -> 0.000000000000   ,  \"τ22\" -> 0.000000000000   ,  \"τN1\" -> 0.000000000000   ,  \"τN2\" -> 0.000000000000   ,  \"σηlogτ1 \" -> 0.000000000000   ,  \"σηlogτS\" -> 0.000000000000   ,  \"σηlogτN\" -> 0.000000000000   ,  \"σlogτ1\" -> 0.000000000000   ,  \"σlogτS\" -> 0.000000000000   ,  \"σlogτN\" -> 0.000000000000   ,  \"σητ1\" -> 0.000000000000   ,  \"σητS \" -> 0.000000000000   ,  \"σητN\" -> 0.000000000000    |>   , \r\"IDS0170_210310_RAW_cal__sam_\" ->   <|    \"ζ\" -> 0.012831327568   ,  \"τ1\" -> 0.013315909415   ,  \"τS\" -> 0.012590836847   ,  \"τN\" -> 0.000065003013   ,  \"τC\" -> 0.005276356243   ,  \"κ0\" -> 0.000000013610   ,  \"mm1\" -> 0.000047406274   ,  \"mm2\" -> 0.013137605540   ,  \"mm3\" -> 0.018225484932   ,  \"T\" -> 1.800000000000   ,  \"B\" -> 12.000000000000   ,  \"θ\" -> 0.000000000000   ,  \"Reoff\" -> 0.000000000000   ,  \"Imoff\" -> 0.000000000000   ,  \"στ1\" -> 0.000000000000   ,  \"στS\" -> 0.000000000000   ,  \"στN\" -> 0.000000000000   ,  \"τ11 \" -> 0.000000000000   ,  \"τ12\" -> 0.000000000000   ,  \"τ22\" -> 0.000000000000   ,  \"τN1\" -> 0.000000000000   ,  \"τN2\" -> 0.000000000000   ,  \"σηlogτ1 \" -> 0.000000000000   ,  \"σηlogτS\" -> 0.000000000000   ,  \"σηlogτN\" -> 0.000000000000   ,  \"σlogτ1\" -> 0.000000000000   ,  \"σlogτS\" -> 0.000000000000   ,  \"σlogτN\" -> 0.000000000000   ,  \"σητ1\" -> 0.000000000000   ,  \"σητS \" -> 0.000000000000   ,  \"σητN\" -> 0.000000000000    |>   , \r\"IDS0171_210310_RAW_cal__ref_\" ->   <|    \"ζ\" -> 0.017116647721   ,  \"τ1\" -> 0.014941878219   ,  \"τS\" -> 0.008392436112   ,  \"τN\" -> 0.000011747084   ,  \"τC\" -> 0.002803142231   ,  \"κ0\" -> 0.000000022439   ,  \"mm1\" -> 0.000035623333   ,  \"mm2\" -> 0.011267010418   ,  \"mm3\" -> 0.014990421338   ,  \"T\" -> 3.100000000000   ,  \"B\" -> 12.000000000000   ,  \"θ\" -> 0.000000000000   ,  \"Reoff\" -> -297959.183673469349   ,  \"Imoff\" -> 0.000000000000   ,  \"στ1\" -> 0.410303910661   ,  \"στS\" -> 0.000232255759   ,  \"στN\" -> 0.188003802712   ,  \"τ11 \" -> 0.000000000000   ,  \"τ12\" -> 0.000000000000   ,  \"τ22\" -> 0.000000000000   ,  \"τN1\" -> 0.000000000000   ,  \"τN2\" -> 0.000000000000   ,  \"σηlogτ1 \" -> 0.000000000000   ,  \"σηlogτS\" -> 0.000000000000   ,  \"σηlogτN\" -> 0.000000000000   ,  \"σlogτ1\" -> 0.000000000000   ,  \"σlogτS\" -> 0.000000000000   ,  \"σlogτN\" -> 0.000000000000   ,  \"σητ1\" -> 0.000000000000   ,  \"σητS \" -> 0.000000000000   ,  \"σητN\" -> 0.000000000000    |>   , \r\"IDS0171_210310_RAW_cal__sam_\" ->   <|    \"ζ\" -> 0.019774146838   ,  \"τ1\" -> 0.013257273421   ,  \"τS\" -> 0.007064131508   ,  \"τN\" -> 0.000028000819   ,  \"τC\" -> 0.006942241845   ,  \"κ0\" -> 0.000000023477   ,  \"mm1\" -> 0.000068886863   ,  \"mm2\" -> 0.012935419574   ,  \"mm3\" -> 0.014427582022   ,  \"T\" -> 3.100000000000   ,  \"B\" -> 12.000000000000   ,  \"θ\" -> 0.000000000000   ,  \"Reoff\" -> 0.000000000000   ,  \"Imoff\" -> 0.000000000000   ,  \"στ1\" -> 0.000000000000   ,  \"στS\" -> 0.000000000000   ,  \"στN\" -> 0.000000000000   ,  \"τ11 \" -> 0.000000000000   ,  \"τ12\" -> 0.000000000000   ,  \"τ22\" -> 0.000000000000   ,  \"τN1\" -> 0.000000000000   ,  \"τN2\" -> 0.000000000000   ,  \"σηlogτ1 \" -> 0.000000000000   ,  \"σηlogτS\" -> 0.000000000000   ,  \"σηlogτN\" -> 0.000000000000   ,  \"σlogτ1\" -> 0.000000000000   ,  \"σlogτS\" -> 0.000000000000   ,  \"σlogτN\" -> 0.000000000000   ,  \"σητ1\" -> 0.000000000000   ,  \"σητS \" -> 0.000000000000   ,  \"σητN\" -> 0.000000000000    |>   , \r\"IDS0172_210310_RAW_cal__ref_\" ->   <|    \"ζ\" -> 0.018105234018   ,  \"τ1\" -> 0.013976020767   ,  \"τS\" -> 0.005494207082   ,  \"τN\" -> 0.000001697310   ,  \"τC\" -> 0.002434353238   ,  \"κ0\" -> 0.000000055294   ,  \"mm1\" -> 0.000030277813   ,  \"mm2\" -> 0.007995449956   ,  \"mm3\" -> 0.013980055263   ,  \"T\" -> 5.500000000000   ,  \"B\" -> 12.000000000000   ,  \"θ\" -> 0.000000000000   ,  \"Reoff\" -> -114285.714285714086   ,  \"Imoff\" -> 0.000000000000   ,  \"στ1\" -> 5.359406809289   ,  \"στS\" -> 0.000541837361   ,  \"στN\" -> 2.799281990955   ,  \"τ11 \" -> 0.000000000000   ,  \"τ12\" -> 0.000000000000   ,  \"τ22\" -> 0.000000000000   ,  \"τN1\" -> 0.000000000000   ,  \"τN2\" -> 0.000000000000   ,  \"σηlogτ1 \" -> 0.000000000000   ,  \"σηlogτS\" -> 0.000000000000   ,  \"σηlogτN\" -> 0.000000000000   ,  \"σlogτ1\" -> 0.000000000000   ,  \"σlogτS\" -> 0.000000000000   ,  \"σlogτN\" -> 0.000000000000   ,  \"σητ1\" -> 0.000000000000   ,  \"σητS \" -> 0.000000000000   ,  \"σητN\" -> 0.000000000000    |>   , \r\"IDS0172_210310_RAW_cal__sam_\" ->   <|    \"ζ\" -> 0.029251354442   ,  \"τ1\" -> 0.014634751206   ,  \"τS\" -> 0.003873958746   ,  \"τN\" -> 0.000007000487   ,  \"τC\" -> 0.006827504775   ,  \"κ0\" -> 0.000000056438   ,  \"mm1\" -> 0.000072018576   ,  \"mm2\" -> 0.010723236476   ,  \"mm3\" -> 0.014661483476   ,  \"T\" -> 5.500000000000   ,  \"B\" -> 12.000000000000   ,  \"θ\" -> 0.000000000000   ,  \"Reoff\" -> 0.000000000000   ,  \"Imoff\" -> 0.000000000000   ,  \"στ1\" -> 0.000000000000   ,  \"στS\" -> 0.000000000000   ,  \"στN\" -> 0.000000000000   ,  \"τ11 \" -> 0.000000000000   ,  \"τ12\" -> 0.000000000000   ,  \"τ22\" -> 0.000000000000   ,  \"τN1\" -> 0.000000000000   ,  \"τN2\" -> 0.000000000000   ,  \"σηlogτ1 \" -> 0.000000000000   ,  \"σηlogτS\" -> 0.000000000000   ,  \"σηlogτN\" -> 0.000000000000   ,  \"σlogτ1\" -> 0.000000000000   ,  \"σlogτS\" -> 0.000000000000   ,  \"σlogτN\" -> 0.000000000000   ,  \"σητ1\" -> 0.000000000000   ,  \"σητS \" -> 0.000000000000   ,  \"σητN\" -> 0.000000000000    |>   , \r\"IDS0181_210310_RAW_cal__ref_\" ->   <|    \"ζ\" -> 0.184661154250   ,  \"τ1\" -> 0.073143653513   ,  \"τS\" -> 0.039056595956   ,  \"τN\" -> 0.118680063461   ,  \"τC\" -> 0.001210341112   ,  \"κ0\" -> 0.000000000912   ,  \"mm1\" -> 0.000184541019   ,  \"mm2\" -> 0.014006042546   ,  \"mm3\" -> 0.247027904072   ,  \"T\" -> 0.179000000000   ,  \"B\" -> 12.000000000000   ,  \"θ\" -> 90.000000000000   ,  \"Reoff\" -> 0.000000000000   ,  \"Imoff\" -> 0.000000000000   ,  \"στ1\" -> 0.002765609964   ,  \"στS\" -> 0.000116033934   ,  \"στN\" -> 0.004164002046   ,  \"τ11 \" -> 0.000000000000   ,  \"τ12\" -> 0.000000000000   ,  \"τ22\" -> 0.000000000000   ,  \"τN1\" -> 0.000000000000   ,  \"τN2\" -> 0.000000000000   ,  \"σηlogτ1 \" -> 0.021708170987   ,  \"σηlogτS\" -> 0.000073917645   ,  \"σηlogτN\" -> 0.039759744455   ,  \"σlogτ1\" -> 0.037810662051   ,  \"σlogτS\" -> 0.002970917754   ,  \"σlogτN\" -> 0.035085943875   ,  \"σητ1\" -> 0.001587814937   ,  \"σητS \" -> 0.000002886972   ,  \"σητN\" -> 0.004718688995    |>   , \r\"IDS0181_210310_RAW_cal__sam_\" ->   <|    \"ζ\" -> 0.161975781729   ,  \"τ1\" -> 0.073089805113   ,  \"τS\" -> 0.045018408115   ,  \"τN\" -> 0.161987434028   ,  \"τC\" -> 0.001482104484   ,  \"κ0\" -> 0.000000001038   ,  \"mm1\" -> 0.000201615809   ,  \"mm2\" -> 0.012976126678   ,  \"mm3\" -> 0.301929942357   ,  \"T\" -> 0.179000000000   ,  \"B\" -> 12.000000000000   ,  \"θ\" -> 90.000000000000   ,  \"Reoff\" -> 0.000000000000   ,  \"Imoff\" -> 0.000000000000   ,  \"στ1\" -> 0.000000000000   ,  \"στS\" -> 0.000000000000   ,  \"στN\" -> 0.000000000000   ,  \"τ11 \" -> 0.000000000000   ,  \"τ12\" -> 0.000000000000   ,  \"τ22\" -> 0.000000000000   ,  \"τN1\" -> 0.000000000000   ,  \"τN2\" -> 0.000000000000   ,  \"σηlogτ1 \" -> 0.000000000000   ,  \"σηlogτS\" -> 0.000000000000   ,  \"σηlogτN\" -> 0.000000000000   ,  \"σlogτ1\" -> 0.000000000000   ,  \"σlogτS\" -> 0.000000000000   ,  \"σlogτN\" -> 0.000000000000   ,  \"σητ1\" -> 0.000000000000   ,  \"σητS \" -> 0.000000000000   ,  \"σητN\" -> 0.000000000000    |>   , \r\"IDS0183_210310_RAW_cal__ref_\" ->   <|    \"ζ\" -> 0.375235391174   ,  \"τ1\" -> 0.100390183494   ,  \"τS\" -> 0.059883674441   ,  \"τN\" -> 0.583268417564   ,  \"τC\" -> 0.001015388210   ,  \"κ0\" -> 0.000000000451   ,  \"mm1\" -> 0.000274513115   ,  \"mm2\" -> 0.008539722831   ,  \"mm3\" -> 0.977076854592   ,  \"T\" -> 0.120000000000   ,  \"B\" -> 12.000000000000   ,  \"θ\" -> 90.000000000000   ,  \"Reoff\" -> 0.000000000000   ,  \"Imoff\" -> 0.000000000000   ,  \"στ1\" -> 0.000375271363   ,  \"στS\" -> 0.000128650872   ,  \"στN\" -> 0.001598463820   ,  \"τ11 \" -> 0.000000000000   ,  \"τ12\" -> 0.000000000000   ,  \"τ22\" -> 0.000000000000   ,  \"τN1\" -> 0.000000000000   ,  \"τN2\" -> 0.000000000000   ,  \"σηlogτ1 \" -> 0.048375297950   ,  \"σηlogτS\" -> 0.002019546500   ,  \"σηlogτN\" -> 0.062171656813   ,  \"σlogτ1\" -> 0.003738128067   ,  \"σlogτS\" -> 0.002148346326   ,  \"σlogτN\" -> 0.002740528669   ,  \"σητ1\" -> 0.004856405038   ,  \"σητS \" -> 0.000120937865   ,  \"σητN\" -> 0.036262763887    |>   , \r\"IDS0183_210310_RAW_cal__sam_\" ->   <|    \"ζ\" -> 0.300863384227   ,  \"τ1\" -> 0.104924004009   ,  \"τS\" -> 0.071070599729   ,  \"τN\" -> 0.992887187112   ,  \"τC\" -> 0.001721587800   ,  \"κ0\" -> 0.000000000548   ,  \"mm1\" -> 0.000392216822   ,  \"mm2\" -> 0.006637384427   ,  \"mm3\" -> 1.483679717825   ,  \"T\" -> 0.120000000000   ,  \"B\" -> 12.000000000000   ,  \"θ\" -> 90.000000000000   ,  \"Reoff\" -> 0.000000000000   ,  \"Imoff\" -> 0.000000000000   ,  \"στ1\" -> 0.000000000000   ,  \"στS\" -> 0.000000000000   ,  \"στN\" -> 0.000000000000   ,  \"τ11 \" -> 0.000000000000   ,  \"τ12\" -> 0.000000000000   ,  \"τ22\" -> 0.000000000000   ,  \"τN1\" -> 0.000000000000   ,  \"τN2\" -> 0.000000000000   ,  \"σηlogτ1 \" -> 0.000000000000   ,  \"σηlogτS\" -> 0.000000000000   ,  \"σηlogτN\" -> 0.000000000000   ,  \"σlogτ1\" -> 0.000000000000   ,  \"σlogτS\" -> 0.000000000000   ,  \"σlogτN\" -> 0.000000000000   ,  \"σητ1\" -> 0.000000000000   ,  \"σητS \" -> 0.000000000000   ,  \"σητN\" -> 0.000000000000    |>   , \r\"IDS0184_210310_RAW_cal__ref_\" ->   <|    \"ζ\" -> 0.249677790636   ,  \"τ1\" -> 0.079352994253   ,  \"τS\" -> 0.040865207813   ,  \"τN\" -> 0.254408476103   ,  \"τC\" -> 0.001065199691   ,  \"κ0\" -> 0.000000000659   ,  \"mm1\" -> 0.000209254261   ,  \"mm2\" -> 0.009370515775   ,  \"mm3\" -> 0.439835388857   ,  \"T\" -> 0.148000000000   ,  \"B\" -> 12.000000000000   ,  \"θ\" -> 90.000000000000   ,  \"Reoff\" -> 0.000000000000   ,  \"Imoff\" -> 0.000000000000   ,  \"στ1\" -> 0.004653512256   ,  \"στS\" -> 0.000201657830   ,  \"στN\" -> 0.014301023172   ,  \"τ11 \" -> 0.000000000000   ,  \"τ12\" -> 0.000000000000   ,  \"τ22\" -> 0.000000000000   ,  \"τN1\" -> 0.000000000000   ,  \"τN2\" -> 0.000000000000   ,  \"σηlogτ1 \" -> 0.022347208648   ,  \"σηlogτS\" -> 0.000103477934   ,  \"σηlogτN\" -> 0.041144706708   ,  \"σlogτ1\" -> 0.058643184169   ,  \"σlogτS\" -> 0.004934707064   ,  \"σlogτN\" -> 0.056212840827   ,  \"σητ1\" -> 0.001773317919   ,  \"σητS \" -> 0.000004228647   ,  \"σητN\" -> 0.010467562133    |>   , \r\"IDS0184_210310_RAW_cal__sam_\" ->   <|    \"ζ\" -> 0.215697702358   ,  \"τ1\" -> 0.095971807771   ,  \"τS\" -> 0.069319630290   ,  \"τN\" -> 0.366712218878   ,  \"τC\" -> 0.001526252261   ,  \"κ0\" -> 0.000000000784   ,  \"mm1\" -> 0.000266752031   ,  \"mm2\" -> 0.013373263674   ,  \"mm3\" -> 0.613940961515   ,  \"T\" -> 0.148000000000   ,  \"B\" -> 12.000000000000   ,  \"θ\" -> 90.000000000000   ,  \"Reoff\" -> 0.000000000000   ,  \"Imoff\" -> 0.000000000000   ,  \"στ1\" -> 0.000000000000   ,  \"στS\" -> 0.000000000000   ,  \"στN\" -> 0.000000000000   ,  \"τ11 \" -> 0.000000000000   ,  \"τ12\" -> 0.000000000000   ,  \"τ22\" -> 0.000000000000   ,  \"τN1\" -> 0.000000000000   ,  \"τN2\" -> 0.000000000000   ,  \"σηlogτ1 \" -> 0.000000000000   ,  \"σηlogτS\" -> 0.000000000000   ,  \"σηlogτN\" -> 0.000000000000   ,  \"σlogτ1\" -> 0.000000000000   ,  \"σlogτS\" -> 0.000000000000   ,  \"σlogτN\" -> 0.000000000000   ,  \"σητ1\" -> 0.000000000000   ,  \"σητS \" -> 0.000000000000   ,  \"σητN\" -> 0.000000000000    |>   , \r\"IDS0185_210310_RAW_cal__ref_\" ->   <|    \"ζ\" -> 0.169435500052   ,  \"τ1\" -> 0.065522222520   ,  \"τS\" -> 0.031885966152   ,  \"τN\" -> 0.085736532349   ,  \"τC\" -> 0.001085511850   ,  \"κ0\" -> 0.000000001071   ,  \"mm1\" -> 0.000153416807   ,  \"mm2\" -> 0.013121484947   ,  \"mm3\" -> 0.190884757967   ,  \"T\" -> 0.197000000000   ,  \"B\" -> 12.000000000000   ,  \"θ\" -> 90.000000000000   ,  \"Reoff\" -> 0.000000000000   ,  \"Imoff\" -> 0.000000000000   ,  \"στ1\" -> 0.000057538627   ,  \"στS\" -> 0.000008322484   ,  \"στN\" -> 0.000057382706   ,  \"τ11 \" -> 0.000000000000   ,  \"τ12\" -> 0.000000000000   ,  \"τ22\" -> 0.000000000000   ,  \"τN1\" -> 0.000000000000   ,  \"τN2\" -> 0.000000000000   ,  \"σηlogτ1 \" -> 0.032785245148   ,  \"σηlogτS\" -> 0.000886609066   ,  \"σηlogτN\" -> 0.045894988103   ,  \"σlogτ1\" -> 0.000878154381   ,  \"σlogτS\" -> 0.000261007731   ,  \"σlogτN\" -> 0.000669291195   ,  \"σητ1\" -> 0.002148162128   ,  \"σητS \" -> 0.000028270387   ,  \"σητN\" -> 0.003934877132    |>   , \r\"IDS0185_210310_RAW_cal__sam_\" ->   <|    \"ζ\" -> 0.139117463690   ,  \"τ1\" -> 0.070330410174   ,  \"τS\" -> 0.040829719954   ,  \"τN\" -> 0.122434321115   ,  \"τC\" -> 0.001436112939   ,  \"κ0\" -> 0.000000001208   ,  \"mm1\" -> 0.000170710071   ,  \"mm2\" -> 0.013785404893   ,  \"mm3\" -> 0.243787328523   ,  \"T\" -> 0.197000000000   ,  \"B\" -> 12.000000000000   ,  \"θ\" -> 90.000000000000   ,  \"Reoff\" -> 0.000000000000   ,  \"Imoff\" -> 0.000000000000   ,  \"στ1\" -> 0.000000000000   ,  \"στS\" -> 0.000000000000   ,  \"στN\" -> 0.000000000000   ,  \"τ11 \" -> 0.000000000000   ,  \"τ12\" -> 0.000000000000   ,  \"τ22\" -> 0.000000000000   ,  \"τN1\" -> 0.000000000000   ,  \"τN2\" -> 0.000000000000   ,  \"σηlogτ1 \" -> 0.000000000000   ,  \"σηlogτS\" -> 0.000000000000   ,  \"σηlogτN\" -> 0.000000000000   ,  \"σlogτ1\" -> 0.000000000000   ,  \"σlogτS\" -> 0.000000000000   ,  \"σlogτN\" -> 0.000000000000   ,  \"σητ1\" -> 0.000000000000   ,  \"σητS \" -> 0.000000000000   ,  \"σητN\" -> 0.000000000000    |>   , \r\"IDS0186_210310_RAW_cal__ref_\" ->   <|    \"ζ\" -> 0.100232193660   ,  \"τ1\" -> 0.049981714900   ,  \"τS\" -> 0.026964705596   ,  \"τN\" -> 0.034498560244   ,  \"τC\" -> 0.001422553924   ,  \"κ0\" -> 0.000000001370   ,  \"mm1\" -> 0.000124145367   ,  \"mm2\" -> 0.014880634319   ,  \"mm3\" -> 0.104023352943   ,  \"T\" -> 0.249000000000   ,  \"B\" -> 12.000000000000   ,  \"θ\" -> 90.000000000000   ,  \"Reoff\" -> 0.000000000000   ,  \"Imoff\" -> 0.000000000000   ,  \"στ1\" -> 0.000091233173   ,  \"στS\" -> 0.000009463067   ,  \"στN\" -> 0.000045871847   ,  \"τ11 \" -> 0.000000000000   ,  \"τ12\" -> 0.000000000000   ,  \"τ22\" -> 0.000000000000   ,  \"τN1\" -> 0.000000000000   ,  \"τN2\" -> 0.000000000000   ,  \"σηlogτ1 \" -> 0.031503726160   ,  \"σηl
